vi "Convert Number to Fault String.vi"(11 "Number":i32) -> (3 "Fault String":string)   [LabVIEW 2020, in "ChromTech Next Gen Compensator Pump.lvlib"]
uses:
  ChromTech Next Gen Compensator Pump.lvlib
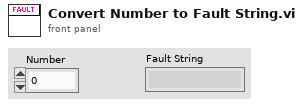
[diagram p1: front panel]
types:
  T1 = typedef "ChromTech Next Gen Compensator Pump.lvlib/Faults.ctl" = enum16{"Upper Pressure Fault", "Lower Pressure Fault", "Motor Stall"}
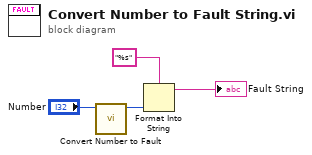
[diagram p0: block diagram]
diagram:
  n1 = call "Convert Number to Fault.vi"("Number"="Number") -> ("Fault"=w2:T1)  [unwired: 10 in]
  n2 = Format Into String(format string="%s", w2) -> (resulting string=→"Fault String":string)  [unwired: 2 in, 1 out]
